vi "CalcExposeWithoutSaturation.vi"(3 "Actual Exposuretime":dbl, 4 "Maximal Intensity that should not be reached":dbl, 5 "Maximal Intensity in Image":sgl) -> (0 "New Exposuretime\nnext smaller":dbl, 1 "New Exposuretime":dbl)   [LabVIEW 2015]
panel:
  # "Calculates best Exposuretime for underexposed Images"
  # "The Lumenera LU105 Camera rounds the exposuretimes \nto the next permitted value. The permitted values are 1/2^x with x element of [3, 4, ... 13]\n\nFor the formular to find the optimal exposuretime T_new=i_max/i_img*T_old it fits \nbetter to use the next smaller exposuretime instead of rounding. \n\nThe formular above doesnt work for a saturated image."
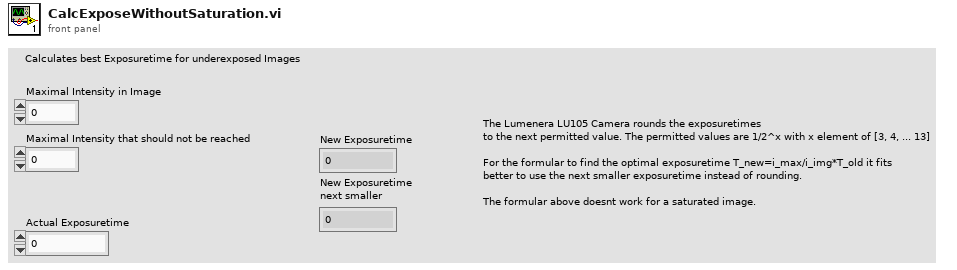
[diagram p1: front panel]
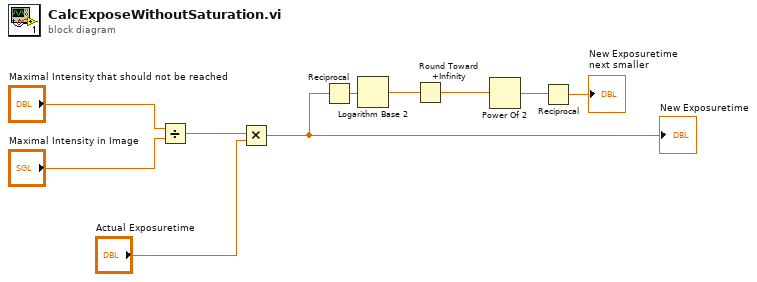
[diagram p0: block diagram]
diagram:
  n1 = Divide(x="Maximal Intensity that should not be reached", y="Maximal Intensity in Image") -> (x/y=w8:dbl)
  n2 = Multiply(x=w8, y="Actual Exposuretime") -> (x*y=w2:dbl)
  "New Exposuretime" <- w2
  n3 = Reciprocal(x=w2) -> (1/x=w6:dbl)
  n4 = Logarithm Base 2(1:w6) -> (0:w5:dbl)
  n5 = Round Toward +Infinity(x=w5) -> (ceil(x): smallest int >= x=w4:dbl)
  n6 = Power Of 2(x=w4) -> (2^x=w3:dbl)
  n7 = Reciprocal(x=w3) -> (1/x=→"New Exposuretime\nnext smaller":dbl)
